vi "averageSpectra.vi"(11 "multipleSpectra":dbl[][][](array[numeric])) -> (1 "meanSpectrum":dbl[](array[numeric]), 2 "frequencies":dbl[](array[numeric]), 3 "spectraPlots":cluster{"Array":dbl[], "Array":dbl[]}[](array[cluster]))   [LabVIEW 2013]
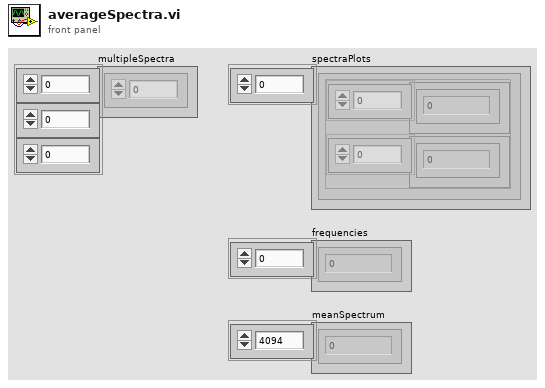
[diagram p1: front panel]
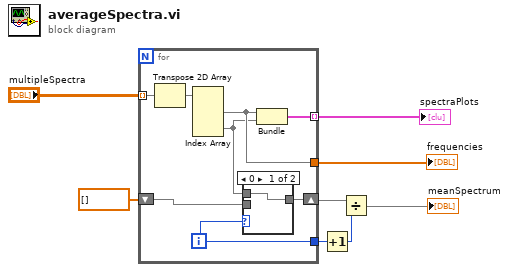
[diagram p0: block diagram]
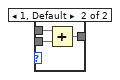
[diagram p2: hidden frame]
diagram:
  n1 = for {
    tunnel: "multipleSpectra" -> [w16] mode=indexing
    tunnel: [w15] -> w4 mode=indexing
    shift-right: [w13] -> w3
    shift-left: dbl[] [] -> [w12]
    tunnel: [w11] -> w7
    tunnel: [w10] -> w5
    i -> [w10]
    n2 = Transpose 2D Array(2D array=w16) -> (transposed array=w14:dbl[][])
    n3 = Index Array(array=w14) -> (element #1=w11:dbl[], element #2=w9:dbl[])  [unwired: 4 in]
    n4 = case shown="0" w10 {
      tunnel: w9 -> [w17 w20]
      tunnel: [w17 w19] -> w13
      tunnel: w12 -> [_ w18]
      frame 0 {
      }
      frame 1, Default {
        n5 = Add(x=w20, y=w18) -> (x+y=w19:dbl[])
      }
    }
    n6 = Bundle(w11, w9) -> (w15:cluster{dbl[], dbl[]})  [unwired: 1 in]
  }
  "frequencies" <- w7
  "spectraPlots" <- w4
  n7 = Increment(x=w5) -> (x+1=w6:i32)
  n8 = Divide(x=w3, y=w6) -> (x/y=→"meanSpectrum":dbl[])
